vi "LabView code.vi"() -> ()   [LabVIEW 2020]
uses:
  System.Speech
  <vilib>/MakerHub/LINX/Public/Peripherals/Digital/Digital Read 1 Chan.vi
  <vilib>/MakerHub/LINX/Public/Peripherals/PWM/PWM Set Duty Cycle 1 Chan.vi
  <vilib>/MakerHub/LINX/Public/Peripherals/Digital/Digital Write.vi
  <vilib>/MakerHub/LINX/Public/Peripherals/Digital/Digital Write 1 Chan.vi
  <vilib>/MakerHub/LINX/Public/Peripherals/Digital/Digital Read N Chans.vi
  <vilib>/MakerHub/LINX/Public/Peripherals/Digital/Digital Write N Chans.vi
  <vilib>/MakerHub/LINX/Private/Local IO/LinxDigitalRead.vi
  <vilib>/MakerHub/LINX/Public/Utilities/Check Channel.vi
  <vilib>/MakerHub/LINX/Private/Local IO/LinxDigitalWrite.vi
  <vilib>/MakerHub/LINX/Public/Utilities/Open Serial.vi
  <vilib>/MakerHub/LINX/Private/Utilties/Generate Error.vi
  <vilib>/MakerHub/LINX/Public/Peripherals/PWM/PWM Set Duty Cycle N Chans.vi
  <vilib>/MakerHub/LINX/Private/Device/Peripheral/Digital/Digital Write.vi
  <vilib>/MakerHub/LINX/LMH-LINX.lvlib
panel:
  out "text":string
  in  "Path":path
  in  "Serial Port":refnum<visa-resource-name>="N/A"
  in  "stop":bool
  out "Sensing indicator":bool
  in  "Motor speed":dbl(slide) scale=0.0..1.0
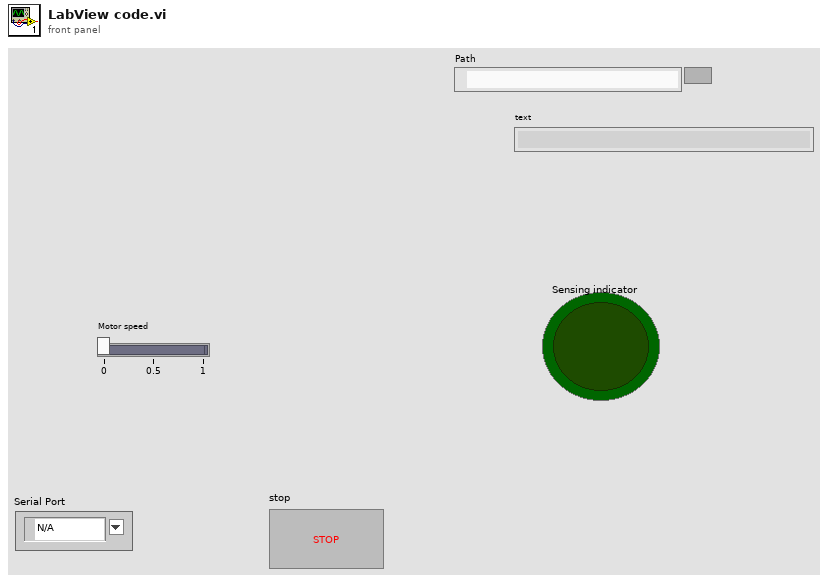
[diagram p1: front panel]
types:
  T1 = typedef "LMH-LINX.lvlib/LINX Ref.ctl" = cluster{"IO":T2, "Interface":T3, "LINX Device Config":T4}
  T2 = typedef "LMH-LINX.lvlib/Platform.ctl" = enum16{"Remote", "Local"}
  T3 = typedef "LMH-LINX.lvlib/Interface.ctl" = enum16{"Serial", "TCP"}
  T4 = typedef "LMH-LINX.lvlib/Device.lvlib/LINX Device Config.ctl" = cluster{"Interface":T3, "COM Port":refnum<visa-resource-name>, "TCP Configuration":T5, "Device Family":u8, "Device ID":u8, "Device Name":string, "TCP Ref":refnum<k5>, "Channels":T6}
  T5 = typedef "LMH-LINX.lvlib/Device.lvlib/TCP Config.ctl" = cluster{"IP Address":string, "Port":u16}
  T6 = typedef "LMH-LINX.lvlib/Channels.ctl" = cluster{"DI":u8[], "DO":u8[], "AI":u8[], "AO":u8[], "PWM":u8[], "QE":u8[], "UART":u8[], "I2C 2":u8[], "SPI":u8[], "CAN":u8[], "Servo":u8[], "AI Ref (V)":dbl, "AI Resolution (Bits)":u8, "AO Ref (V)":dbl, "AO Resolution (Bits)":u8}
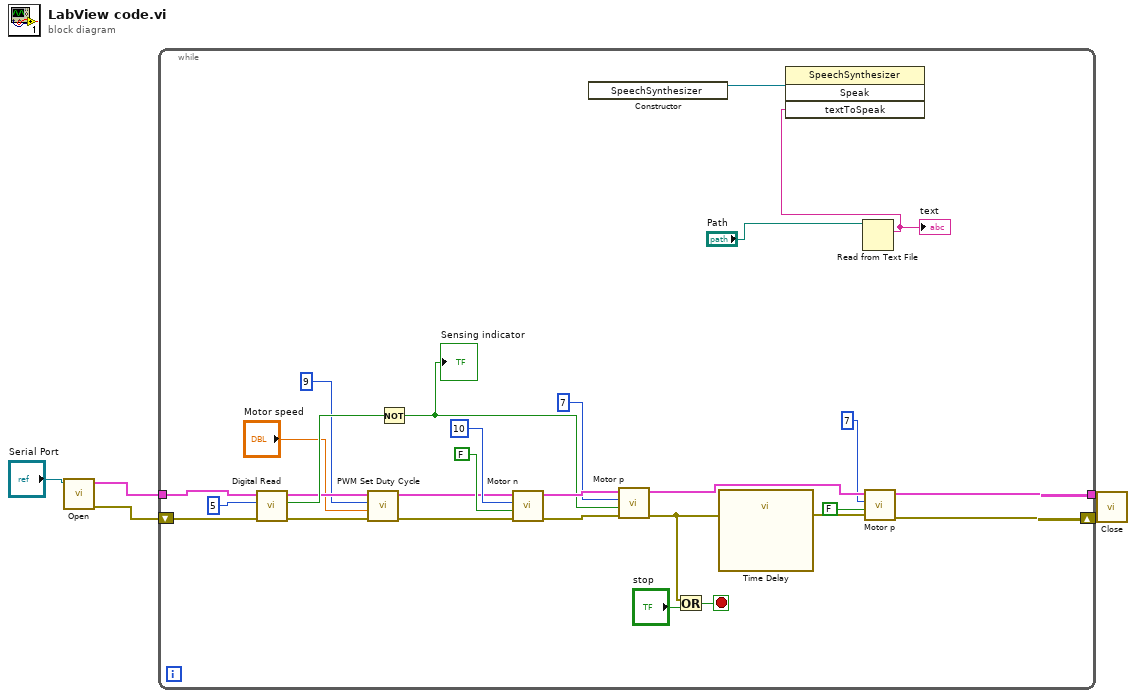
[diagram p0: block diagram]
diagram:
  n1 = call-poly <vilib>:"Open.vi"("Serial Port"="Serial Port") -> ("Error Out"=w5:errorcluster, "LINX Resource"=w3:T1)  [unwired: 8 in, 1 out]
  n2 = while {
    shift-right: [w13] -> w1
    shift-left: w5 -> [w32]
    tunnel: w3 -> [w27]
    tunnel: [w14] -> w2
    stop <- w29 stop-if-true
    n3 = call-poly <vilib>:"Digital Read.vi"("Error In"=w32, "DI Channel"=u8 5, "LINX Resource"=w27) -> ("Error Out"=w20:errorcluster, "DI Value"=w33:bool, "LINX Resource"=w21:T1)  [unwired: 6 in]
    n4 = call-poly <vilib>:"PWM Set Duty Cycle.vi"("Error In"=w20, "Duty Cycle (0-1)"="Motor speed", "PWM Channel"=u8 9, "LINX Resource"=w21) -> ("Error Out"=w18:errorcluster, "LINX Resource"=w19:T1)  [unwired: 6 in]
    n5 = Not(x=w33) -> (.not. x?=w22:bool)
    "Sensing indicator" <- w22
    n6 = call-poly "Motor n"("Error In"=w18, "Output Value"=FALSE, "DO Channel"=u8 10, "LINX Resource"=w19) -> ("Error Out"=w30:errorcluster, "LINX Resource"=w31:T1)  [unwired: 6 in]
    n7 = constructor class="SpeechSynthesizer"() -> (reference out=w8:refnum<k24>)  [unwired: 3 in, 2 out]
    n8 = call-poly "Motor p"("Error In"=w30, "Output Value"=w22, "DO Channel"=u8 7, "LINX Resource"=w31) -> ("Error Out"=w15:errorcluster, "LINX Resource"=w11:T1)  [unwired: 6 in]
    n9 = Or(x=w15, y="stop") -> (x .or. y?=w29:bool)
    n10 = call "Time Delay"("error in (no error)"=w15) -> ("error out"=w12:errorcluster)  [unwired: 10 in]
    n11 = Read from Text File(file (use dialog)="Path") -> (text=w6:string)  [unwired: 3 in, 3 out]
    "text" <- w6
    n12 = invoke class="SpeechSynthesizer" method="Speak"(reference=w8, "textToSpeak"=w6) -> ()  [unwired: 2 in, 4 out]
    n13 = call-poly "Motor p"("Error In"=w12, "Output Value"=FALSE, "DO Channel"=u8 7, "LINX Resource"=w11) -> ("Error Out"=w13:errorcluster, "LINX Resource"=w14:T1)  [unwired: 6 in]
  }
  n14 = call <vilib>:"Close.vi"("Error In"=w1, "LINX Resource"=w2) -> ()  [unwired: 9 in, 1 out]
